vi "main.vi"() -> ()   [LabVIEW 2016]
uses:
  <resource>/objmgr/IMAQImage.rc
panel:
  in  "Número de passos":u32
  in  "Window":cluster{"Rw":i32, "Rh":i32}={"Rw"=30, "Rh"=20}
  out "pontos quentes":cluster{i32, i32}[](array[cluster])
  out "initialized array":sgl[][](array[numeric])
  out "Array":T1(array[cluster])
  out "Image":T2(plugin-control)
  in  "threshold":sgl
  in  "K":u16
  in  "# máximo de iterações":i32=25
  in  "sigma (mu=0)":sgl format="%#_13g"
  in  "Temperatures":cluster{"Ts":sgl, "Tp":sgl, "Tb":sgl}
  in  "target size":cluster{"sx":i32, "sy":i32}
  in  "target positions":cluster{"x":i32, "y":i32}[](array[cluster])
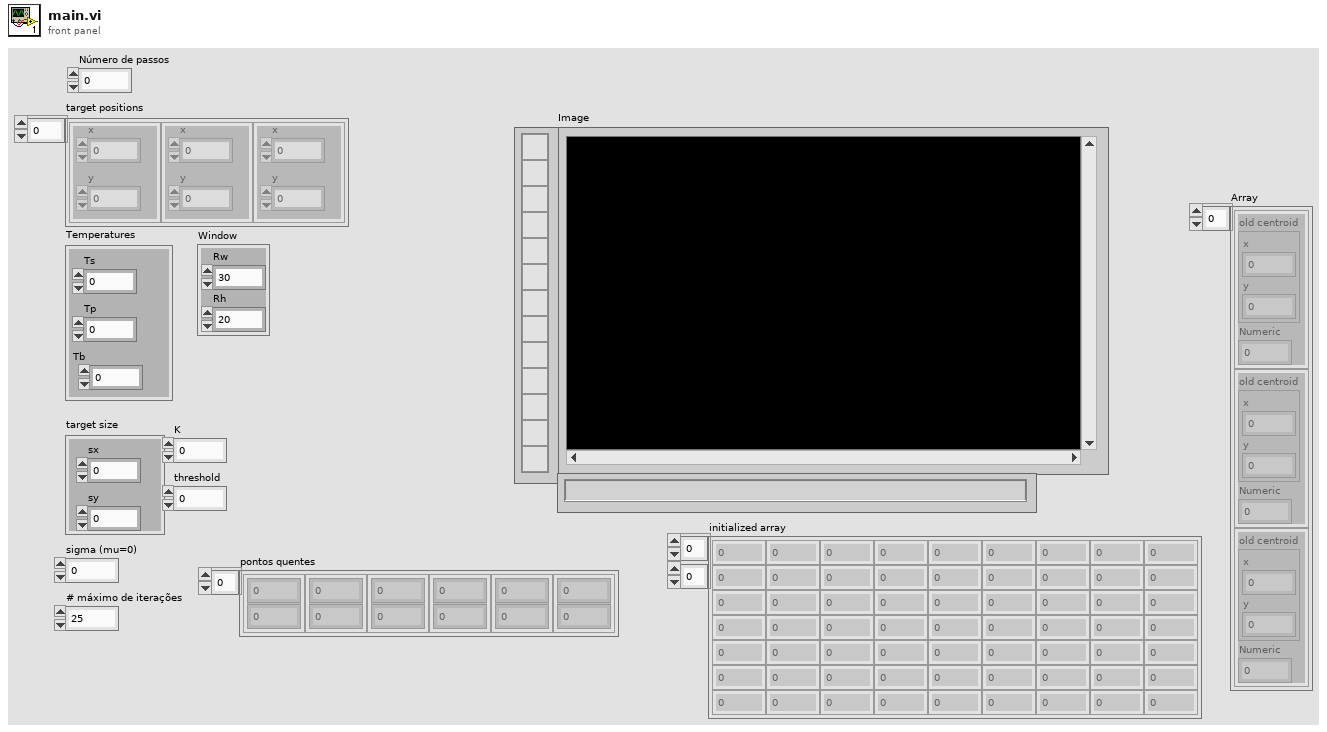
[diagram p1: front panel]
types:
  T1 = cluster{"old centroid":cluster{"x":dbl, "y":dbl}, "Numeric":i32}[]
  T2 = typedef "IMAQ Image.ctl" = refnum<image>
  T3 = cluster{"old centroid":cluster{"x":dbl, "y":dbl}, "Numeric":i32}
  T4 = typedef "Image Type" = u32
  T5 = cluster{"Desired Font (Application)":enum16{"User-specified Font", "Application Font", "System Font", "Dialog Font"}, "[User-specified Font]":cluster{"Font Name":string, "Size":i16, "Strikeout?":bool, "Italic?":bool, "Underline?":bool, "Outline?":bool, "Shadow?":bool, "Bold?":bool, "Rotation Angle":dbl}, "Horizontal Alignment":i16, "Vertical Alignment":i16}
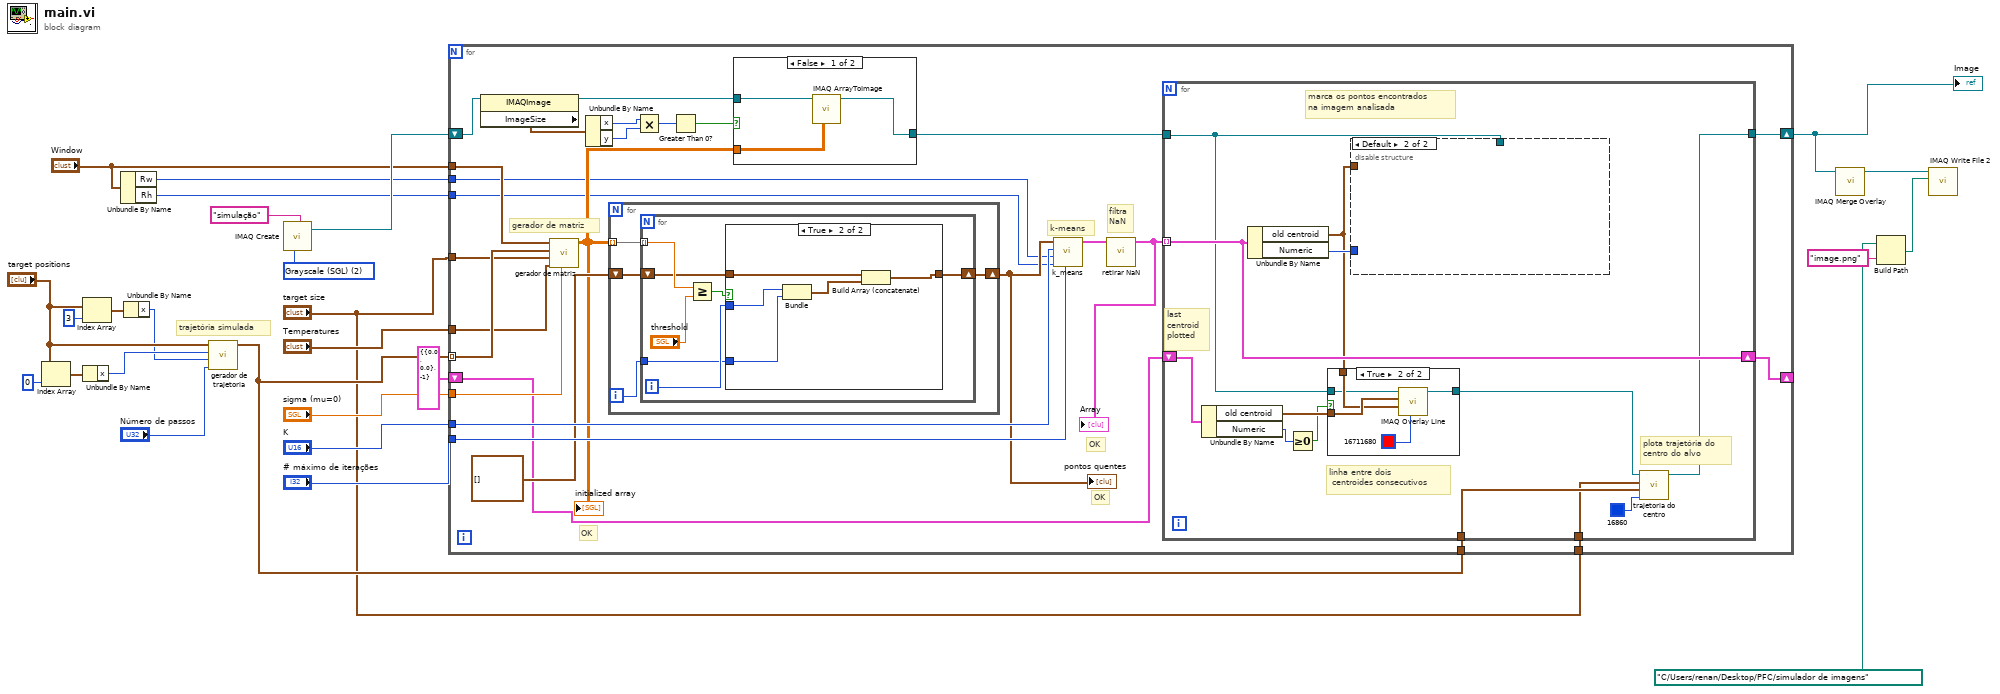
[diagram p0: block diagram]
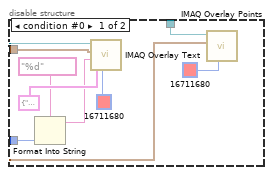
[diagram p4: hidden frame]
diagram:
  w25 = T4 2 items=["Grayscale (U8)", "Grayscale (I16)", "Grayscale (SGL)", "Complex (CSG)", "RGB (U32)", "HSL (U32)", "RGB (U64)", "Grayscale (U16)"] ("Image Type")
  # "trajetória simulada"
  n1 = Index Array(array="target positions", index=0) -> (element=w10:cluster{"x":i32, "y":i32})
  n2 = Index Array(array="target positions", index=3) -> (element=w8:cluster{"x":i32, "y":i32})
  n3 = Unbundle By Name(w10) -> ("x"=w6:i32)
  n4 = Unbundle By Name("Window") -> ("Rw"=w12:i32, "Rh"=w13:i32)
  n5 = Unbundle By Name(w8) -> ("x"=w5:i32)
  n6 = call "gerador de trajetoria.vi"("passar pelos\npontos:"="target positions", "x inicial"=w6, "x final"=w5, "Número de passos"="Número de passos") -> ("pontos\ninterpolados"=w3:cluster{"X":dbl, "Y":dbl}[])  [unwired: 6 in]
  n7 = call "IMAQ Create"("Image Name"="simulação", "Image Type"=w25) -> ("New Image"=w20:T2)  [unwired: 3 in, 1 out]
  n8 = for {
    tunnel: w3 -> [w53] mode=indexing
    tunnel: "Window" -> [w49]
    tunnel: "target size" -> [w52]
    tunnel: "Temperatures" -> [w51]
    tunnel: "sigma (mu=0)" -> [w50]
    tunnel: "# máximo de iterações" -> [w48]
    tunnel: "K" -> [w47]
    shift-right: [w46] -> w4
    shift-left: w20 -> [w42]
    tunnel: w12 -> [w33]
    tunnel: w13 -> [w34]
    tunnel: w3 -> [w32]
    tunnel: "target size" -> [w31]
    shift-right: [w28] -> _
    shift-left: T3 {"old centroid"={"x"=0.0, "y"=0.0}, "Numeric"=-1} ("centroide (ponto, índice) 2") -> [w27]
    # "filtra\nNaN"
    # "OK"
    # "OK"
    # "OK"
    # "gerador de matriz"
    # "k-means"
    n9 = property class="IMAQImage"(reference=w42) -> (reference out=w41:T2, "ImageSize"=w40:cluster{"x":i32, "y":i32})  [unwired: 1 in, 1 out]
    n10 = call "gerador de matriz.vi"("sigma"=w50, "Temperatures"=w51, "target size"=w52, "target position"=w53, "Window"=w49) -> ("initialized array"=w35:sgl[][])  [unwired: 5 in, 1 out]
    "initialized array" <- w35
    n11 = Unbundle By Name(w40) -> ("x"=w39:i32, "y"=w38:i32)
    n12 = for {
      tunnel: w35 -> [w88] mode=indexing
      shift-right: [w85] -> w45
      shift-left: cluster{i32, i32}[] [] -> [w87]
      i -> [w86]
      n13 = for {
        tunnel: w88 -> [w95] mode=indexing
        tunnel: w86 -> [w90]
        shift-right: [w89] -> w85
        shift-left: w87 -> [w92]
        i -> [w91]
        n14 = Greater Or Equal?(x=w95, y="threshold") -> (x >= y?=w93:bool)
        n15 = case shown="True" w93 {
          tunnel: w92 -> [w96 w101]
          tunnel: w91 -> [_ w97]
          tunnel: w90 -> [_ w98]
          tunnel: [w96 w100] -> w89
          frame False {
          }
          frame True {
            n16 = Bundle(w97, w98) -> (w99:cluster{i32, i32})  [unwired: 1 in]
            n17 = Build Array (concatenate)(w101, w99) -> (w100:cluster{i32, i32}[])
          }
        }
      }
    }
    "pontos quentes" <- w45
    n18 = Multiply(x=w39, y=w38) -> (x*y=w37:i32)
    n19 = Greater Than 0?(x=w37) -> (x > 0?=w36:bool)
    n20 = case shown="False" w36 {
      tunnel: w35 -> [w56 _]
      tunnel: [w55 w57] -> w43
      tunnel: w41 -> [w54 w57]
      frame False {
        n21 = call "IMAQ ArrayToImage"("Image Pixels (Float)"=w56, "Image"=w54) -> ("Image Out"=w55:T2)  [unwired: 8 in, 1 out]
      }
      frame True {
      }
    }
    n22 = call "k_means.vi"("# máximo de iterações"=w48, "altura (pixels)"=w34, "largura (pixels)"=w33, "K"=w47, "point array"=w45) -> ("Array"=w30:T1)  [unwired: 5 in, 1 out]
    n23 = call "retirar NaN.vi"("Array"=w30) -> ("Array Out"=w29:T1)  [unwired: 10 in]
    "Array" <- w29
    n24 = for {
      tunnel: w29 -> [w67] mode=indexing
      tunnel: [w60] -> w46
      tunnel: w43 -> [w62]
      shift-right: [w67] -> w28
      shift-left: w27 -> [w68]
      tunnel: w32 -> [w65]
      tunnel: w31 -> [w64]
      # "plota trajetória do\ncentro do alvo"
      # "last\ncentroid\nplotted"
      # "linha entre dois\n centroides consecutivos"
      # "marca os pontos encontrados\nna imagem analisada"
      n25 = Unbundle By Name(w68) -> ("old centroid"=w69:cluster{"x":dbl, "y":dbl}, "Numeric"=w59:i32)
      n26 = Unbundle By Name(w67) -> ("old centroid"=w66:cluster{"x":dbl, "y":dbl}, "Numeric"=w70:i32)
      n27 = Greater Or Equal To 0?(x=w59) -> (x >= 0?=w58:bool)
      n28 = case shown="True" w58 {
        tunnel: w69 -> [_ w76]
        tunnel: w66 -> [_ w75]
        tunnel: w62 -> [w71 w73]
        tunnel: [w71 w72] -> w61
        frame False {
        }
        frame True {
          n29 = call "IMAQ Overlay Line"("Color"=u32 16711680, "End Point"=w75, "Start Point"=w76, "Image"=w73) -> ("Image Out"=w72:T2)  [unwired: 6 in, 1 out]
        }
      }
      n30 = disable-structure shown="Default" {
        disable-tunnel: w70 -> [w81 _]
        disable-tunnel: w66 -> [w78 _]
        disable-tunnel: w62 -> [w77 _]
        frame condition #0 {
          n31 = Format Into String(format string="%d", w81) -> (resulting string=w80:string)  [unwired: 2 in, 1 out]
          n32 = call "IMAQ Overlay Text"("Text Color (black)"=u32 16711680, "Font, Size & Style"=T5 {"Desired Font (Application)"=enum."Application Font", "[User-specified Font]"={"Font Name"="", "Size"=32, "Strikeout?"=FALSE, "Italic?"=FALSE, "Underline?"=FALSE, "Outline?"=FALSE, "Shadow?"=FALSE, "Bold?"=TRUE, "Rotation Angle"=0.0}, "Horizontal Alignment"=0, "Vertical Alignment"=0}, "String"=w80, "Origin"=w78, "Image"=w77) -> ()  [unwired: 5 in, 2 out]
          n33 = call "IMAQ Overlay Points"("Color"=u32 16711680, "Point"=w78, "Image"=w77) -> ()  [unwired: 7 in, 2 out]
        }
        frame condition #1 (active) {
        }
      }
      n34 = call "trajetoria do centro.vi"("Color"=u32 16860, "pontos\ninterpolados"=w65, "target size"=w64, "Refnum in"=w61) -> ("Refnum out"=w60:T2)  [unwired: 7 in]
    }
  }
  "Image" <- w4
  n35 = call "IMAQ Merge Overlay"("Image Src"=w4) -> ("Image Dst Out"=w19:T2)  [unwired: 9 in, 1 out]
  n36 = Build Path(base path=path "C:/Users/renan/Desktop/PFC/simulador de imagens", name or relative path="image.png") -> (appended path=w18:path)
  n37 = call-poly "IMAQ Write File 2"("File Path"=w18, "Image"=w19) -> ()  [unwired: 8 in, 2 out]
